vi "del_bats.vi"(10 "Endereço de saída (.mat)":path=path "G:/ATP_SIMULACOES_v2/dados_brutos", 11 "Diretório de trabalho":path=path "C:/ATP/ATPDraw/Projects_Flavio") -> ()   [LabVIEW 2020]
panel:
  out "deleted path":path
  out "filenames":string[](array[string])
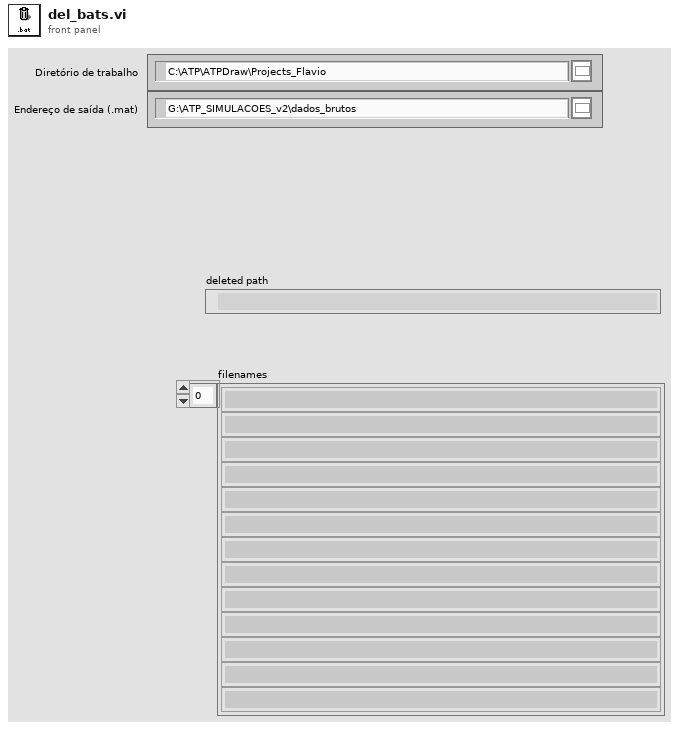
[diagram p1: front panel]
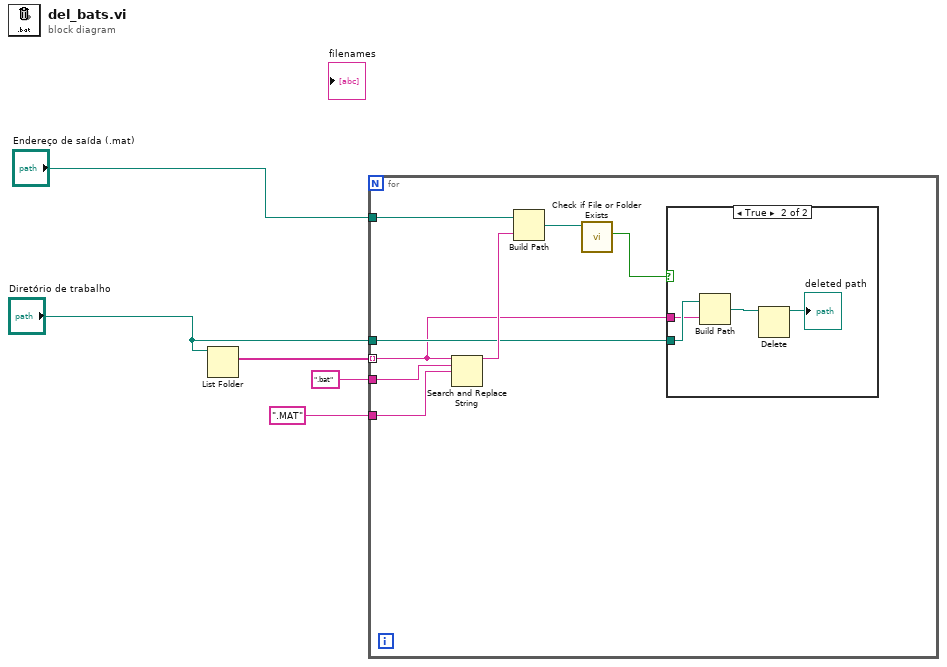
[diagram p0: block diagram]
diagram:
  n1 = List Folder(path="Diretório de trabalho") -> (filenames=w3:string[])  [unwired: 3 in, 3 out]
  n2 = for {
    tunnel: w3 -> [w6] mode=indexing
    tunnel: ".MAT" ("pattern") -> [w12]
    tunnel: ".bat" ("pattern") -> [w13]
    tunnel: "Endereço de saída (.mat)" -> [w11]
    tunnel: "Diretório de trabalho" -> [w8]
    n3 = Search and Replace String(input string=w6, search string=w13, replace string=w12) -> (result string=w10:string)  [unwired: 5 in, 3 out]
    n4 = Build Path(base path=w11, name or relative path=w10) -> (appended path=w9:path)
    n5 = call <vilib>:"Check if File or Folder Exists.vi"("path"=w9) -> ("file or folder exists?"=w7:bool)  [unwired: 8 in, 2 out]
    n6 = case shown="True" w7 {
      tunnel: w8 -> [_ w15]
      tunnel: w6 -> [_ w14]
      frame False {
      }
      frame True {
        n7 = Build Path(base path=w15, name or relative path=w14) -> (appended path=w16:path)
        n8 = Delete(path (use dialog)=w16) -> (deleted path=→"deleted path":path)  [unwired: 4 in, 2 out]
      }
    }
  }
